vi "Calculate_Candidates_Tracks-1.vi"(4 "error IN":errorcluster, 6 "[IN] Start Pos of\nMissed Pr Dot":i32, 7 "[IN] Before Pro\ncessing Tracks":T1(array[cluster])) -> (0 "error OUT":errorcluster, 3 "[OUT] Indicies of \ngroup candidates":i32[](array[numeric]))   [LabVIEW 2017]
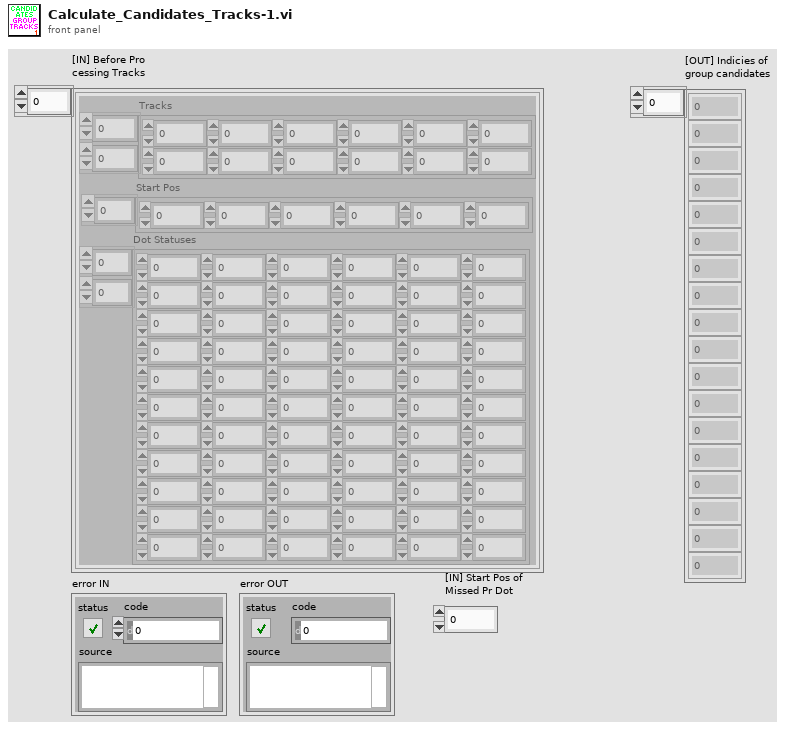
[diagram p1: front panel]
types:
  T1 = cluster{"Tracks":dbl[][], "Start Pos":i32[], "Dot Statuses":i16[][]}[]
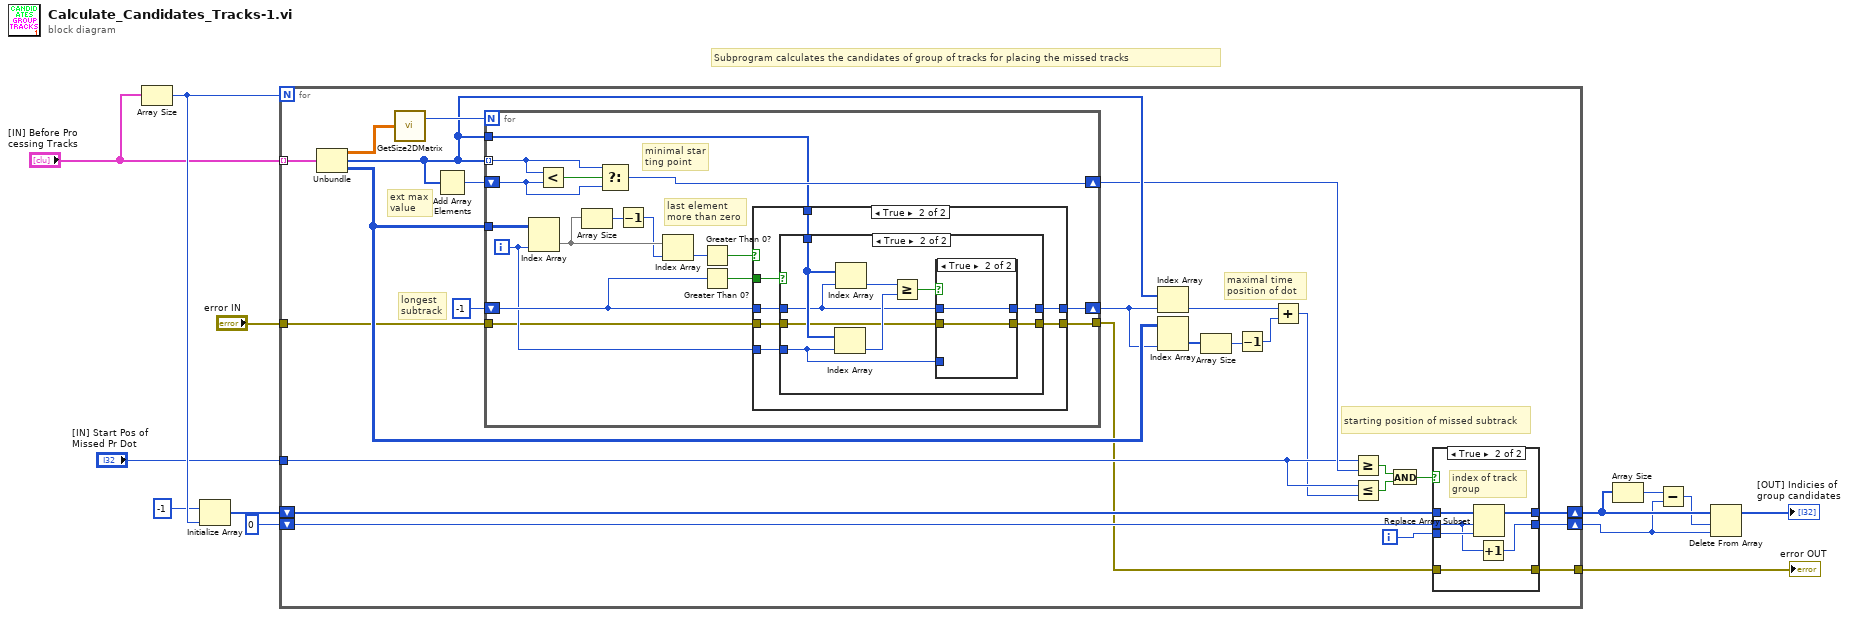
[diagram p0: block diagram]
diagram:
  # "Subprogram calculates the candidates of group of tracks for placing the missed tracks"
  n1 = Array Size(array="[IN] Before Pro\ncessing Tracks") -> (size(s)=w13:i32)
  n2 = Initialize Array(-1 ("size(s)"), w13) -> (w10:i32[])
  n3 = for {
    N: w13 -> [_]
    tunnel: "[IN] Before Pro\ncessing Tracks" -> [w39] mode=indexing
    shift-right: [w17] -> w5
    shift-left: w10 -> [w20]
    shift-right: [w16] -> w3
    shift-left: 0 -> [w19]
    tunnel: "[IN] Start Pos of\nMissed Pr Dot" -> [w26]
    tunnel: "error IN" -> [w21]
    tunnel: [w14] -> w6
    i -> [w18]
    # "starting position of missed subtrack"
    # "maximal time\nposition of dot"
    # "longest \nsubtrack"
    # "ext max \nvalue"
    n4 = Unbundle(w39) -> ("Tracks"=w38:dbl[][], "Start Pos"=w34:i32[], "Dot Statuses"=w32:i16[][])
    n5 = call "GetSize2DMatrix.vi"("Array IN (2D)"=w38) -> ("# Cols"=w37:i32)  [unwired: 1 out]
    n6 = Add Array Elements(numeric array=w34) -> (sum=w36:i32)
    n7 = for {
      N: w37 -> [_]
      tunnel: w34 -> [w64] mode=indexing
      shift-right: [w62] -> w27
      shift-left: w36 -> [w63]
      tunnel: w32 -> [w61]
      shift-right: [w51] -> w31
      shift-left: -1 -> [w53]
      tunnel: w34 -> [w54]
      tunnel: w21 -> [w50]
      tunnel: [w49] -> w15
      i -> [w52]
      # "last element \nmore than zero"
      # "minimal star\nting point"
      n8 = Index Array(array=w61, index (col)=w52) -> (element=w59:i16[])  [unwired: 1 in]
      n9 = Less?(x=w64, y=w63) -> (x < y?=w65:bool)
      n10 = Array Size(array=w59) -> (size(s)=w60:i32)
      n11 = Select(t=w64, s=w65, f=w63) -> (s? t:f=w62:i32)
      n12 = Decrement(x=w60) -> (x-1=w58:i32)
      n13 = Index Array(array=w59, index=w58) -> (element=w57:i16)
      n14 = Greater Than 0?(x=w57) -> (x > 0?=w56:bool)
      n15 = Greater Than 0?(x=w53) -> (x > 0?=w55:bool)
      n16 = case shown="True" w56 {
        tunnel: w55 -> [_ w74]
        tunnel: w54 -> [_ w73]
        tunnel: w53 -> [w67 w72]
        tunnel: w52 -> [_ w71]
        tunnel: [w67 w70] -> w51
        tunnel: w50 -> [w66 w69]
        tunnel: [w66 w68] -> w49
        frame False {
        }
        frame True {
          n17 = case shown="True" w74 {
            tunnel: w73 -> [_ w85]
            tunnel: w72 -> [_ w81]
            tunnel: w71 -> [w76 w79]
            tunnel: [w76 w80] -> w70
            tunnel: w69 -> [w75 w78]
            tunnel: [w75 w77] -> w68
            frame False {
            }
            frame True {
              n18 = Index Array(array=w85, index=w79) -> (element=w83:i32)
              n19 = Index Array(array=w85, index=w81) -> (element=w84:i32)
              n20 = Greater Or Equal?(x=w84, y=w83) -> (x >= y?=w82:bool)
              n21 = case shown="True" w82 {
                tunnel: w81 -> [_ w89]
                tunnel: [w87 w89] -> w80
                tunnel: w79 -> [w87 _]
                tunnel: [w86 w88] -> w77
                tunnel: w78 -> [w86 w88]
                frame False {
                }
                frame True {
                }
              }
            }
          }
        }
      }
    }
    n22 = Index Array(array=w34, index=w31) -> (element=w33:i32)
    n23 = Index Array(array=w32, index (col)=w31) -> (element=w30:i16[])  [unwired: 1 in]
    n24 = Array Size(array=w30) -> (size(s)=w29:i32)
    n25 = Decrement(x=w29) -> (x-1=w28:i32)
    n26 = Add(x=w33, y=w28) -> (x+y=w25:i32)
    n27 = Greater Or Equal?(x=w26, y=w27) -> (x >= y?=w24:bool)
    n28 = Less Or Equal?(x=w26, y=w25) -> (x <= y?=w23:bool)
    n29 = And(x=w24, y=w23) -> (x .and. y?=w22:bool)
    n30 = case shown="True" w22 {
      tunnel: w20 -> [w42 w48]
      tunnel: w19 -> [w41 w45]
      tunnel: w18 -> [_ w47]
      tunnel: [w42 w46] -> w17
      tunnel: [w41 w44] -> w16
      tunnel: w15 -> [w40 w43]
      tunnel: [w40 w43] -> w14
      frame False {
      }
      frame True {
        # "index of track \ngroup"
        n31 = Replace Array Subset(array=w48, new element=w47, index=w45) -> (w46:i32[])
        n32 = Increment(x=w45) -> (x+1=w44:i32)
      }
    }
  }
  "error OUT" <- w6
  n33 = Array Size(array=w5) -> (size(s)=w4:i32)
  n34 = Subtract(x=w4, y=w3) -> (x-y=w2:i32)
  n35 = Delete From Array(array=w5, length=w2, index=w3) -> (array with subset deleted=→"[OUT] Indicies of \ngroup candidates":i32[])  [unwired: 1 out]
